vi "Generate Pulse Train.vi"() -> ()   [LabVIEW 2015]
uses:
  <vilib>/DAQmx/create/channels.llb/DAQmx Create Channel (CO-Pulse Generation-Ticks).vi
  <vilib>/DAQmx/configure/timing.llb/DAQmx Timing (Implicit).vi
panel:
  in  "stop":bool
  in  "Interval (ms)":dbl=131.35355 format="%#_12g"
  in  "Pulse width (us)":dbl=1000.0
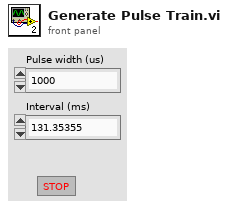
[diagram p1: front panel]
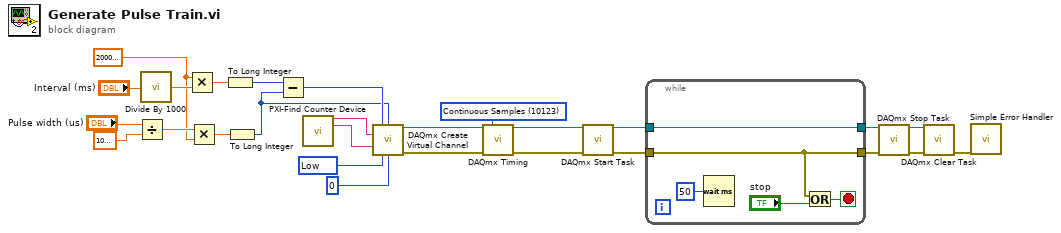
[diagram p0: block diagram]
diagram:
  w24 = 10214 items=["High"=10192, "Low"=10214] ("idle state")
  w15 = 20000000.0
  w27 = 10123 items=["Finite Samples"=10178, "Continuous Samples"=10123] ("sample mode")
  n1 = Divide(x="Pulse width (us)", y=1000000.0) -> (x/y=w16:dbl)
  n2 = call "Divide By 1000.vi"("X"="Interval (ms)") -> ("X/1000"=w21:dbl)
  n3 = Multiply(x=w15, y=w21) -> (x*y=w20:dbl)
  n4 = Multiply(x=w16, y=w15) -> (x*y=w17:dbl)
  n5 = To Long Integer(number=w20) -> (32bit integer=w14:i32)
  n6 = To Long Integer(number=w17) -> (32bit integer=w1:i32)
  n7 = Subtract(x=w14, y=w1) -> (x-y=w2:i32)
  n8 = call "PXI-Find Counter Device.vi"() -> ("Counter Channel"=w4:tag, "RefClk.Src"=w3:tag)  [unwired: 12 in, 2 out]
  n9 = call-poly <vilib>:"DAQmx Create Virtual Channel.vi"("high ticks"=w2, "low ticks"=w1, "counter"=w4, "source of ticks"=w3, "idle state"=w24, "initial delay"=u32 0) -> ("task out"=w26:refnum<k21>, "error out"=w25:errorcluster)  [unwired: 8 in]
  n10 = call-poly <vilib>:"DAQmx Timing.vi"("task/channels in"=w26, "sample mode"=w27, "error in"=w25) -> ("task out"=w13:refnum<k21>, "error out"=w12:errorcluster)  [unwired: 11 in]
  n11 = call <vilib>:"DAQmx Start Task.vi"("task/channels in"=w13, "error in"=w12) -> ("task out"=w10:refnum<k21>, "error out"=w11:errorcluster)  [unwired: 12 in]
  n12 = while {
    tunnel: w11 -> [w28]
    tunnel: w10 -> [w30]
    tunnel: [w30] -> w9
    tunnel: [w28] -> w8
    stop <- w29 stop-if-true
    n13 = Wait (ms)(milliseconds to wait=u32 50) -> ()  [unwired: 1 out]
    n14 = Or(x=w28, y="stop") -> (x .or. y?=w29:bool)
  }
  n15 = call <vilib>:"DAQmx Stop Task.vi"("task/channels in"=w9, "error in"=w8) -> ("task out"=w7:refnum<k21>, "error out"=w6:errorcluster)  [unwired: 12 in]
  n16 = call <vilib>:"DAQmx Clear Task.vi"("task in"=w7, "error in"=w6) -> ("error out"=w5:errorcluster)  [unwired: 13 in]
  n17 = call <vilib>:"Simple Error Handler.vi"("error in (no error)"=w5) -> ()  [unwired: 4 in, 5 out]
